vi "leapSeconds LUT.vi"() -> (1 "Leap Seconds":i64[](array[numeric]), 3 "UTC Time":i64[](array[numeric]))   [LabVIEW 2013, in "Epoch.lvclass"]
uses:
  Epoch.lvclass
  <vilib>/regexp/Match Regular Expression.xnode
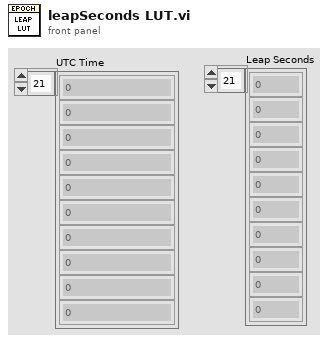
[diagram p1: front panel]
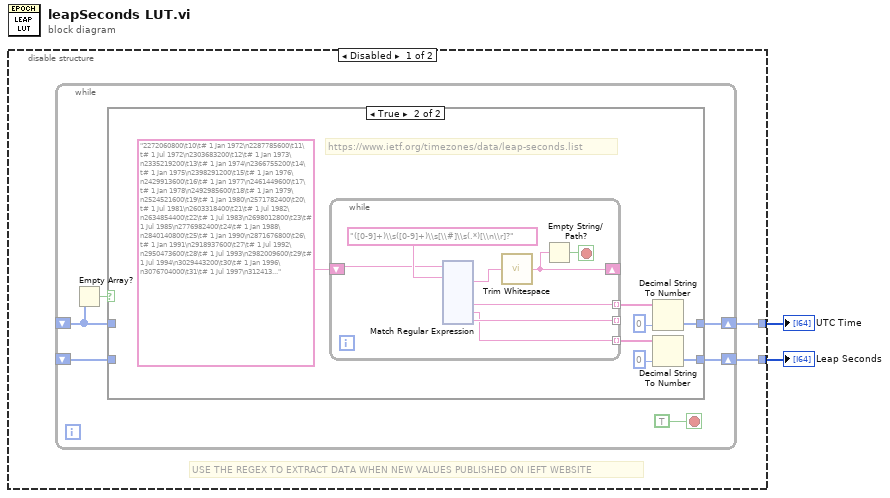
[diagram p0: block diagram]
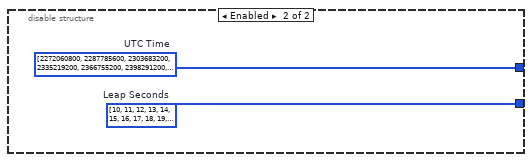
[diagram p3: hidden frame]
diagram:
  n1 = disable-structure shown="Disabled" {
    disable-tunnel: [w4 w147] -> w2
    disable-tunnel: [w3 w146] -> w1
    frame Disabled {
      # "USE THE REGEX TO EXTRACT DATA WHEN NEW VALUES PUBLISHED ON IEFT WEBSITE"
      n2 = while {
        shift-right: [w9] -> w3
        shift-left: _ -> [w6]
        shift-right: [w10] -> w4
        shift-left: _ -> [w5]
        stop <- TRUE stop-if-true
        n3 = Empty Array?(array=w6) -> (empty?=w7:bool)
        n4 = case shown="True" w7 {
          tunnel: [w11 w14] -> w10
          tunnel: [w12 w13] -> w9
          tunnel: w6 -> [w12 _]
          tunnel: w5 -> [w11 _]
          frame False {
          }
          frame True {
            # "https://www.ietf.org/timezones/data/leap-seconds.list"
            n5 = while {
              shift-right: [w25] -> _
              shift-left: "2272060800\t10\t# 1 Jan 1972\n2287785600\t11\t# 1 Jul 1972\n2303683200\t12\t# 1 Jan 1973\n2335219200\t13\t# 1 Jan 1974\n2366755200\t14\t# 1 Jan 1975\n2398291200\t15\t# 1 Jan 1976\n2429913600\t16\t# 1 Jan 1977\n2461449600\t17\t# 1 Jan 1978\n2492985600\t18\t# 1 Jan 1979\n2524521600\t19\t# 1 Jan 1980\n2571782400\t20\t# 1 Jul 1981\n2603318400\t21\t# 1 Jul 1982\n2634854400\t22\t# 1 Jul 1983\n2698012800\t23\t# 1 Jul 1985\n2776982400\t24\t# 1 Jan 1988\n2840140800\t25\t# 1 Jan 1990\n2871676800\t26\t# 1 Jan 1991\n2918937600\t27\t# 1 Jul 1992\n2950473600\t28\t# 1 Jul 1993\n2982009600\t29\t# 1 Jul 1994\n3029443200\t30\t# 1 Jan 1996\n3076704000\t31\t# 1 Jul 1997\n3124137600\t32\t# 1 Jan 1999\n3345062400\t33\t# 1 Jan 2006\n3439756800\t34\t# 1 Jan 2009\n3550089600\t35\t# 1 Jul 2012\n3644697600\t36\t# 1 Jul 2015\n3692217600\t37\t# 1 Jan 2017" -> [w23]
              tunnel: [w22] -> w18 mode=indexing
              tunnel: [w21] -> _ mode=indexing
              tunnel: [w20] -> w15 mode=indexing
              stop <- w26 stop-if-true
              n6 = xnode "Match Regular Expression"("input string"=w23, "regular expression"="([0-9]+)\\s([0-9]+)\\s[\\#]\\s(.*)[\\n\\r]?") -> ("after match"=w27:string, "submatch 1"=w22:string, "submatch 2"=w20:string, "submatch 3"=w21:string)  [unwired: 4 in, 4 out]
              n7 = call <vilib>:"Trim Whitespace.vi"("string"=w27) -> ("trimmed string"=w25:string)  [unwired: 1 in]
              n8 = Empty String/Path?(string/path=w25) -> (empty?=w26:bool)
            }
            n9 = Decimal String To Number(string=w18, default (0L)=i64 0 ("Epoch Time (s)")) -> (number=w13:i64[])  [unwired: 1 in, 1 out]
            n10 = Decimal String To Number(string=w15, default (0L)=i64 0 ("Epoch Time (s)")) -> (number=w14:i64[])  [unwired: 1 in, 1 out]
          }
        }
      }
    }
    frame Enabled {
      w147 = i64[] [10, 11, 12, 13, 14, 15, 16, 17, 18, 19, 20, 21, 22, 23, 24, 25, 26, 27, 28, 29, 30, 31, 32, 33, 34, 35, 36, 37]  # Leap Seconds
      w146 = i64[] [2272060800, 2287785600, 2303683200, 2335219200, 2366755200, 2398291200, 2429913600, 2461449600, 2492985600, 2524521600, 2571782400, 2603318400, 2634854400, 2698012800, 2776982400, 2840140800, 2871676800, 2918937600, 2950473600, 2982009600, 3029443200, 3076704000, 3124137600, 3345062400, 3439756800, 3550089600, 3644697600, 3692217600]  # UTC Time
    }
  }
  "Leap Seconds" <- w2
  "UTC Time" <- w1
